vi "SAOMM-Graph-Guiding.vi"(0 "SNR Data":T1 {"Flux" format="%.6f"; "SNRtreshold" format="%.6f"; "SNR" format="%.6f"}, 1 "TimeStamp":dbl, 2 "DataLenght (seconds)":dbl, 5 "Centroids Data":T2 {"CenY" format="%.6f"; "CenX" format="%.6f"}, 7 "SNR IN":cluster{dbl[], dbl[]}[](array[cluster]) {"?" format="%.1f"}, 9 "Flux IN":cluster{dbl[], dbl[]}[](array[cluster]), 11 "Centroids IN":cluster{dbl[], dbl[]}[](array[cluster])) -> (8 "SNR OUT":cluster{dbl[], dbl[]}[](array[cluster]) {"?" format="%.3f"}, 10 "Flux OUT":cluster{dbl[], dbl[]}[](array[cluster]), 15 "Centroids OUT":cluster{dbl[], dbl[]}[](array[cluster]))   [LabVIEW 2019]
panel:
  out "ErrY":dbl
  out "ErrX":dbl
  out "Treshold Index":dbl
  out "CurrentTimeStamp":dbl format="%.3f"
  out "TimeStampTreshold":dbl format="%.3f"
  # "Ce VI actualise les graphiques de guidage à partir des informations contenues dans les trame\n'emtHexapodCommandLogging' ou 'emtFalconProcessed'\nDe la façon que les choses sont faites actuellement, ont a les graphiques suivants:\n\n1- SNR, SNRtreshold\n2- Flux de l'étoile (pourrait être normalisé ?!?)\n3- CenX, CenY (ROIX + CenX - PixX, ROIY + CenY - PixY)"
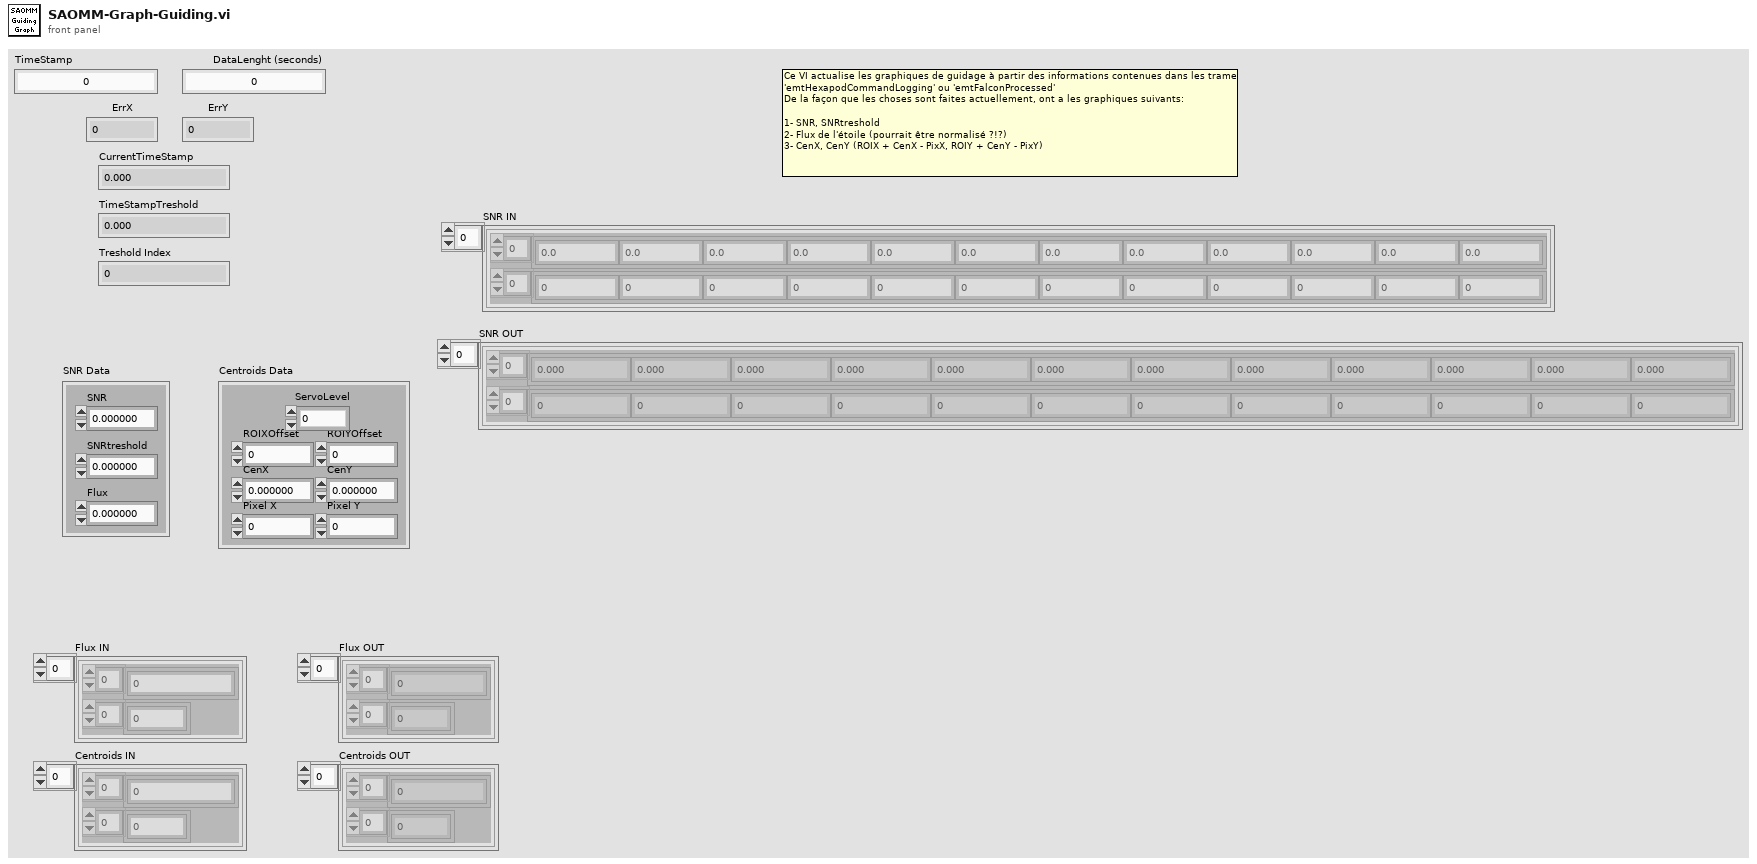
[diagram p1: front panel]
types:
  T1 = cluster{"SNR":dbl, "SNRtreshold":dbl, "Flux":dbl}
  T2 = cluster{"ServoLevel":u16, "ROIXOffset":u16, "CenX":dbl, "Pixel X":dbl, "ROIYOffset":u16, "CenY":dbl, "Pixel Y":dbl}
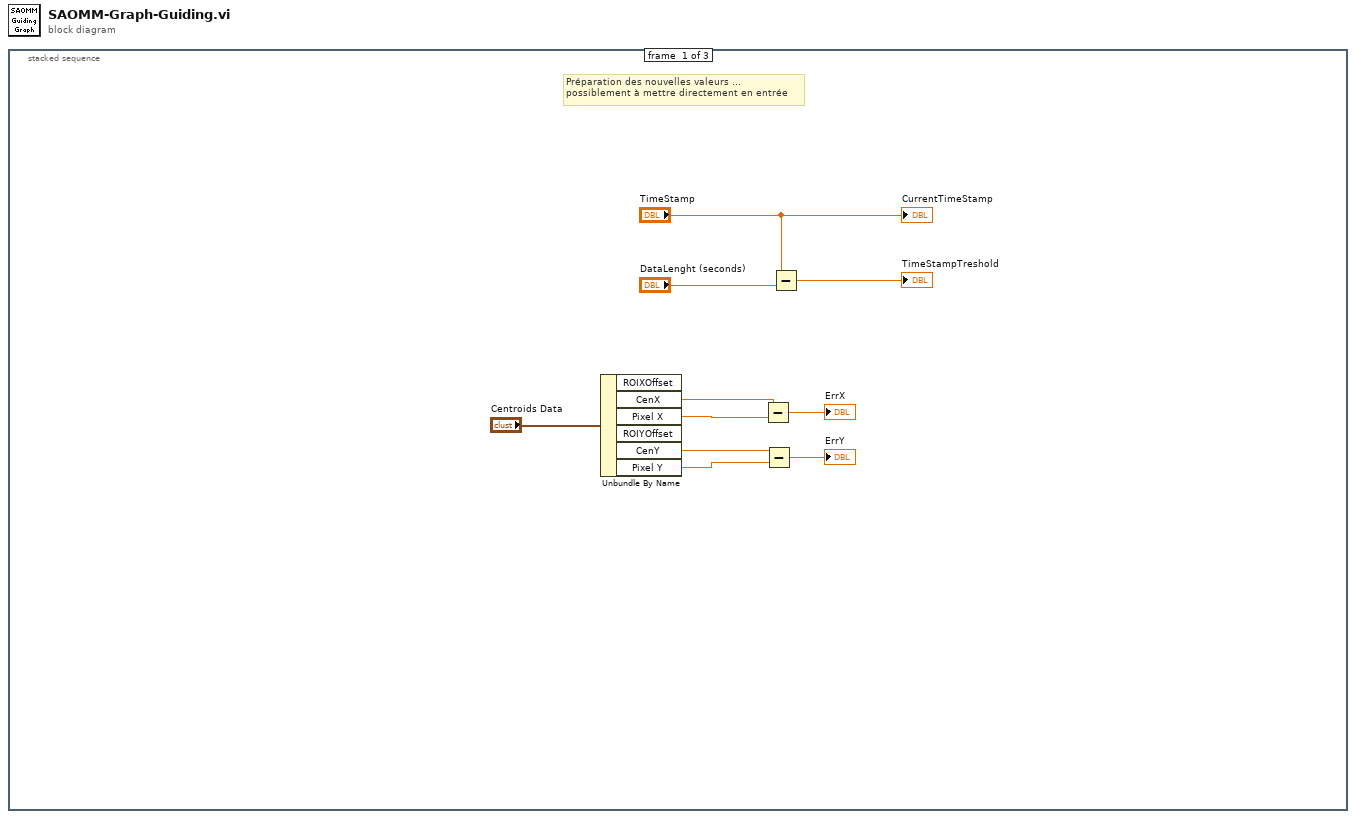
[diagram p0: block diagram]
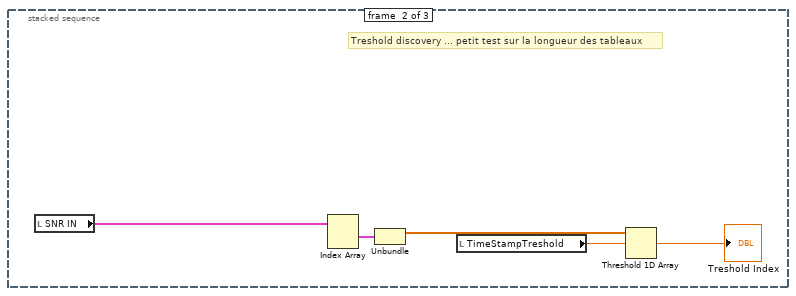
[diagram p2: hidden frame]
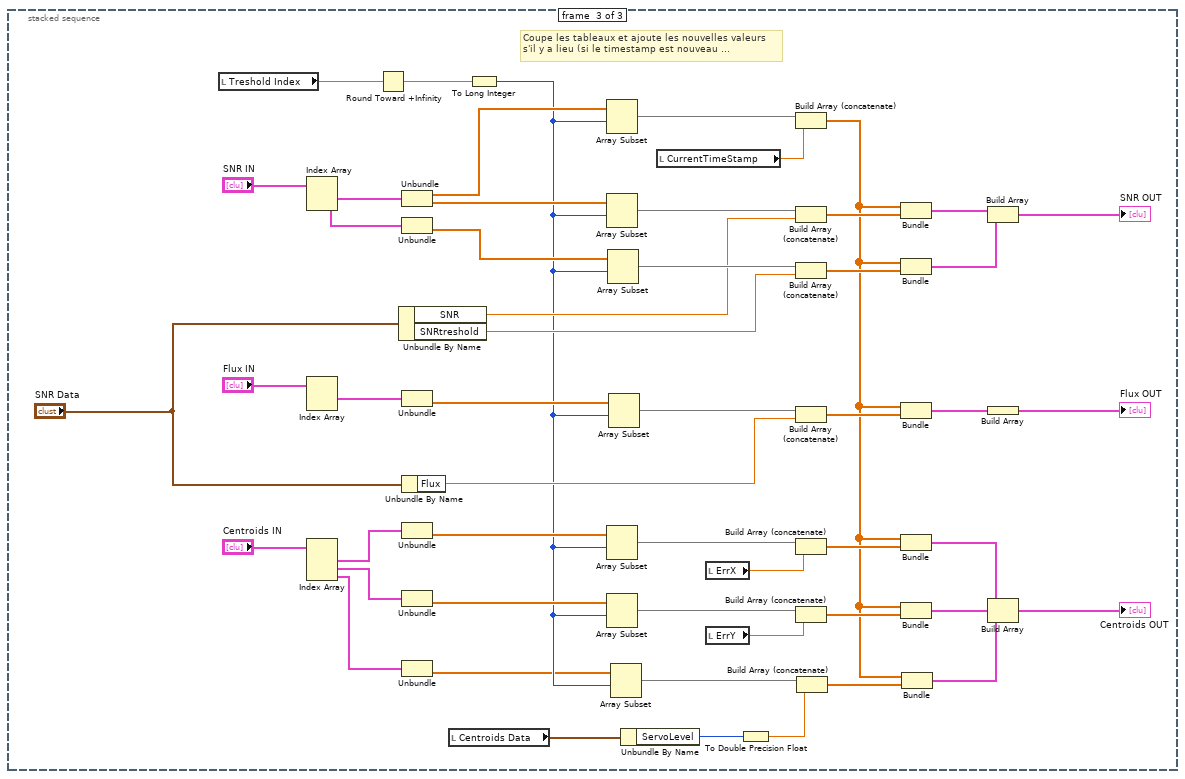
[diagram p3: hidden frame]
diagram:
  n1 = stacked-sequence {
    frame #0 {
      # "Préparation des nouvelles valeurs ...\npossiblement à mettre directement en entrée"
      n2 = Unbundle By Name("Centroids Data") -> ("CenX"=w3:dbl, "Pixel X"=w7:dbl, "CenY"=w2:dbl, "Pixel Y"=w6:dbl)  [unwired: 2 out]
      n3 = Subtract(x=w3, y=w7) -> (x-y=→"ErrX":dbl)
      n4 = Subtract(x=w2, y=w6) -> (x-y=→"ErrY":dbl)
      n5 = Subtract(x="TimeStamp", y="DataLenght (seconds)") -> (x-y=→"TimeStampTreshold":dbl)
      "CurrentTimeStamp" <- "TimeStamp"
    }
    frame #1 {
      # "Treshold discovery ... petit test sur la longueur des tableaux"
      n6 = local read "SNR IN"() -> (w11:cluster{dbl[], dbl[]}[])
      n7 = Index Array(array=w11) -> (element #1=w15:cluster{dbl[], dbl[]})  [unwired: 2 in, 1 out]
      n8 = Unbundle(w15) -> (w14:dbl[])  [unwired: 1 out]
      n9 = local read "TimeStampTreshold"() -> (w13:dbl)
      n10 = Threshold 1D Array(2:w13, 3:w14) -> (0:→"Treshold Index":dbl)  [unwired: 1 in]
    }
    frame #2 {
      # "Coupe les tableaux et ajoute les nouvelles valeurs\ns'il y a lieu (si le timestamp est nouveau ..."
      n11 = local read "Treshold Index"() -> (w60:dbl)
      n12 = Index Array(array="SNR IN") -> (element #1=w52:cluster{dbl[], dbl[]}, element #2=w47:cluster{dbl[], dbl[]})  [unwired: 2 in]
      n13 = Index Array(array="Flux IN") -> (element #1=w38:cluster{dbl[], dbl[]})  [unwired: 2 in, 1 out]
      n14 = Index Array(array="Centroids IN") -> (element #1=w67:cluster{dbl[], dbl[]}, element #2=w66:cluster{dbl[], dbl[]}, element #3=w24:cluster{dbl[], dbl[]})  [unwired: 3 in]
      n15 = Round Toward +Infinity(x=w60) -> (ceil(x): smallest int >= x=w59:dbl)
      n16 = Unbundle By Name("SNR Data") -> ("SNR"=w27:dbl, "SNRtreshold"=w32:dbl)
      n17 = Unbundle(w52) -> (w42:dbl[], w58:dbl[])
      n18 = Unbundle(w47) -> (w43:dbl[])  [unwired: 1 out]
      n19 = Unbundle(w38) -> (w26:dbl[])  [unwired: 1 out]
      n20 = Unbundle By Name("SNR Data") -> ("Flux"=w31:dbl)
      n21 = Unbundle(w67) -> (w57:dbl[])  [unwired: 1 out]
      n22 = Unbundle(w66) -> (w50:dbl[])  [unwired: 1 out]
      n23 = Unbundle(w24) -> (w22:dbl[])  [unwired: 1 out]
      n24 = local read "Centroids Data"() -> (w25:T2)
      n25 = To Long Integer(number=w59) -> (32bit integer=w23:i32)
      n26 = Array Subset(array=w42, index=w23) -> (w54:dbl[])  [unwired: 1 in]
      n27 = Array Subset(array=w58, index=w23) -> (w56:dbl[])  [unwired: 1 in]
      n28 = Array Subset(array=w57, index=w23) -> (w55:dbl[])  [unwired: 1 in]
      n29 = Array Subset(array=w50, index=w23) -> (w51:dbl[])  [unwired: 1 in]
      n30 = Array Subset(array=w43, index=w23) -> (w46:dbl[])  [unwired: 1 in]
      n31 = Array Subset(array=w26, index=w23) -> (w40:dbl[])  [unwired: 1 in]
      n32 = Array Subset(array=w22, index=w23) -> (w21:dbl[])  [unwired: 1 in]
      n33 = Unbundle By Name(w25) -> ("ServoLevel"=w20:u16)
      n34 = local read "CurrentTimeStamp"() -> (w61:dbl)
      n35 = local read "ErrX"() -> (w29:dbl)
      n36 = local read "ErrY"() -> (w30:dbl)
      n37 = To Double Precision Float(number=w20) -> (double precision float=w19:dbl)
      n38 = Build Array (concatenate)(w54, w61) -> (w17:dbl[])
      n39 = Build Array (concatenate)(w56, w27) -> (w62:dbl[])
      n40 = Build Array (concatenate)(w46, w32) -> (w45:dbl[])
      n41 = Build Array (concatenate)(w40, w31) -> (w41:dbl[])
      n42 = Build Array (concatenate)(w55, w29) -> (w48:dbl[])
      n43 = Build Array (concatenate)(w51, w30) -> (w49:dbl[])
      n44 = Build Array (concatenate)(w21, w19) -> (w16:dbl[])
      n45 = Bundle(w17, w62) -> (w65:cluster{dbl[], dbl[]})  [unwired: 1 in]
      n46 = Bundle(w17, w45) -> (w44:cluster{dbl[], dbl[]})  [unwired: 1 in]
      n47 = Bundle(w17, w41) -> (w36:cluster{dbl[], dbl[]})  [unwired: 1 in]
      n48 = Bundle(w17, w48) -> (w64:cluster{dbl[], dbl[]})  [unwired: 1 in]
      n49 = Bundle(w17, w49) -> (w63:cluster{dbl[], dbl[]})  [unwired: 1 in]
      n50 = Bundle(w17, w16) -> (w18:cluster{dbl[], dbl[]})  [unwired: 1 in]
      n51 = Build Array(w65, w44) -> (→"SNR OUT":cluster{dbl[], dbl[]}[])
      n52 = Build Array(w36) -> (→"Flux OUT":cluster{dbl[], dbl[]}[])
      n53 = Build Array(w64, w63, w18) -> (→"Centroids OUT":cluster{dbl[], dbl[]}[])
    }
  }
